vi "PH_SHS_Analysis.pack Zernickes.vi"(1 "SHS Zernicke Dataset":T1 {"State" items=["no info", "off/false/out", "on/true/in", "Failure", "Alarm", "Status 1", "Status 2", "Status 3"]; "Zernicke Coefficients"."2nd Spherical" scale=-2.0..2.0 scale format="%.2f"; "Zernicke Coefficients"."2nd Coma y" scale=-2.0..2.0 scale format="%.2f"; "Zernicke Coefficients"."2nd Coma x" scale=-2.0..2.0 scale format="%.2f"; "Zernicke Coefficients"."2nd Astig 45°" scale=-2.0..2.0 scale format="%.2f"; "Zernicke Coefficients"."2nd Astig 0°" scale=-2.0..2.0 scale format="%.2f"; "Zernicke Coefficients"."Trefoil 30°" scale=-2.0..2.0 scale format="%.2f"; "Zernicke Coefficients"."Trefoil 0°" scale=-2.0..2.0 scale format="%.2f"; "Zernicke Coefficients"."Spherical" scale=-2.0..2.0 scale format="%.2f"; "Zernicke Coefficients"."Coma y" scale=-2.0..2.0 scale format="%.2f"; "Zernicke Coefficients"."Coma x" scale=-2.0..2.0 scale format="%.2f"; "Zernicke Coefficients"."Astig 45°" scale=-2.0..2.0 scale format="%.2f"; "Zernicke Coefficients"."Astig 0°" scale=-2.0..2.0 scale format="%.2f"; "Zernicke Coefficients"."Defocus" scale=-2.0..2.0 scale format="%.2f"; "Zernicke Coefficients"."Tilt y" scale=-2.0..2.0 scale format="%.2f"; "Zernicke Coefficients"."Tilt x" scale=-2.0..2.0 scale format="%.2f"}) -> (0 "DIM Service Array":dbl[](array[numeric]))   [LabVIEW 2014, in "PH_SHS_Analysis.lvlib"]
doc: "This VI packs the Data published as DIM service \"<SHS Anaylzer Instance>_Zernikes\" by the SHS Analyzer."
uses:
  PH_SHS_Analysis.lvlib
  PH_SHS_Analysis.Zernike Dataset.ctl
  PH_Basics/PH_StatusHandler/PH_StatusHandler.Status.ctl
  PH_SHS_Analysis.Zernike Coefficients.ctl
  PH_Basics/PH_StatusHandler/PH_StatusHandler.lvlib
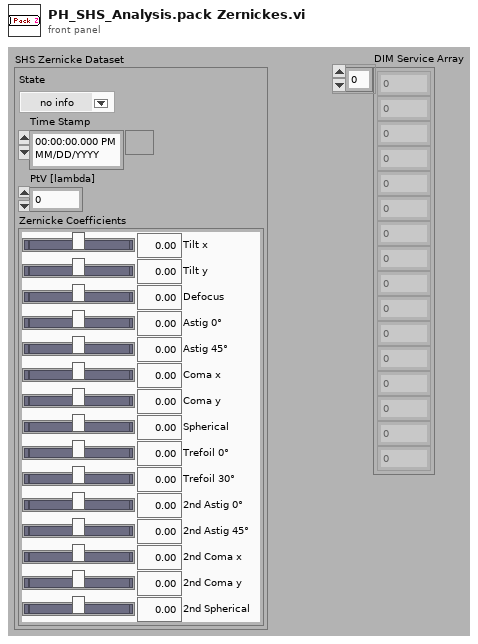
[diagram p1: front panel]
types:
  T1 = typedef "PH_SHS_Analysis.lvlib/PH_SHS_Analysis.Zernike Dataset.ctl" = cluster{"State":T2, "Time Stamp":timestamp, "PtV [lambda]":dbl, "Zernicke Coefficients":T3}
  T2 = typedef "PH_StatusHandler.lvlib/PH_StatusHandler.Status.ctl" = i16
  T3 = typedef "PH_SHS_Analysis.lvlib/PH_SHS_Analysis.Zernike Coefficients.ctl" = cluster{"Tilt x":dbl, "Tilt y":dbl, "Defocus":dbl, "Astig 0°":dbl, "Astig 45°":dbl, "Coma x":dbl, "Coma y":dbl, "Spherical":dbl, "Trefoil 0°":dbl, "Trefoil 30°":dbl, "2nd Astig 0°":dbl, "2nd Astig 45°":dbl, "2nd Coma x":dbl, "2nd Coma y":dbl, "2nd Spherical":dbl}
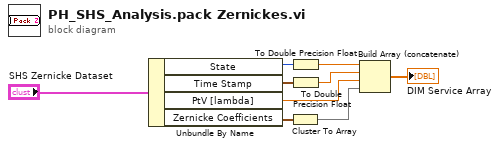
[diagram p0: block diagram]
diagram:
  n1 = Unbundle By Name("SHS Zernicke Dataset") -> ("State"=w5:T2, "Time Stamp"=w6:timestamp, "PtV [lambda]"=w9:dbl, "Zernicke Coefficients"=w3:T3)
  n2 = Cluster To Array(cluster=w3) -> (array=w4:dbl[])
  n3 = To Double Precision Float(number=w5) -> (double precision float=w8:dbl)
  n4 = To Double Precision Float(number=w6) -> (double precision float=w7:dbl)
  n5 = Build Array (concatenate)(w8, w7, w9, w4) -> (→"DIM Service Array":dbl[])
